vi "Lockin.DAQ.TestLauncher.vi"() -> ()   [LabVIEW 2019, in "Instrument.DAQ.lvclass"]
uses:
  Instrument.DAQ.lvclass
  <vilib>/JKI/JKI SMO/SMO/SMO.lvclass
  <vilib>/JKI/JKI SMO/SMO/Typedefs/SMOState --Enum.ctl
  Typedefs/Set State-enum.ctl
  C:/Program Files (x86)/National Instruments/LabVIEW 2019/vi.lib/JKI/JKI SMO/SMO/SMO.lvclass
  Instrument.Lockin/Instrument.Lockin.lvclass
  Instrument.Lockin/Typedefs/Results Type--Enum.ctl
  Typedefs/AO.Function--Enum.ctl
  Typedefs/AO.Channel--Cluster--Array.ctl
  Typedefs/REF.Channel--Cluster--Array.ctl
  Typedefs/DAQ.Sampling--Cluster.ctl
  Typedefs/DAQ.Sample Mode--Ring.ctl
  Typedefs/Get State-enum.ctl
  Typedefs/REF.Channel--Cluster.ctl
  Typedefs/AO.Channel--Cluster.ctl
  Typedefs/DAQ.AO.Range--enum.ctl
  Typedefs/DAQ.AI.Range--enum.ctl
  Typedefs/DAQ.AI.Coupling--enum.ctl
  Typedefs/DAQ.Configuration--Cluster.ctl
panel:
  out "DAQ state":T1=enum."created"
  in  "Tab Control 2":T2(tab)=enum."AI"
  out "AO":waveform(dbl)[](graph)
  out "AI":waveform(dbl)[](graph)
  out "WFM 3":waveform(dbl)[](graph)
  out "REF":waveform(dbl)[](graph)
  out "Results":dbl[](graph)
  in  "Reset DAQ":bool
  in  "Stop DAQ":bool
  in  "Start DAQ":bool
  in  "Tab Control":enum32{"Output", "REF", "DAQ"}(tab)=enum."REF"
  in  "Channels: AO":T3=[{"Enable?"=TRUE, "Channel"=0, "Amplitude"=0.1, "Offset"=0.0, "Frequency"=15.0, "Phase"=0.0, "Function"=enum."Sine", "Sweeping?"=FALSE}, {"Enable?"=TRUE, "Channel"=0, "Amplitude"=0.05, "Offset"=0.0, "Frequency"=13.0, "Phase"=0.0, "Function"=enum."Sine", "Sweeping?"=FALSE}] {"Phase" format="%.3g"; "Frequency" min=0.0001 max=10000.0 format="%.3g"; "Offset" format="%.3p"; "Amplitude" min=0.0 max=10.0 format="%.3p"}
  in  "Channels: Lockin":T6=[{"Enable?"=TRUE, "Channel"=1, "Frequency"=13.0, "Phase"=0.0, "TC"=1e-05, "Roll-Off"=1}] {"Roll-Off" min=1; "TC" min=0.0001 format="%#_3p"; "Phase" format="%.3g"; "Frequency" min=0.0001 max=10000.0 format="%.3g"; "Channel" min=1}
  in  "Gain":dbl[](array[numeric])=[1.0, 1.0]
  in  "sampling":T8={"Fs"=204789.0, "#s"=15753}
  in  "sample mode":T9=10123 items=["Finite Samples"=10178, "Continuous Samples"=10123]
  in  "New Ch []":T10[](array[typedef]) {"AI.Coupling" items=["AC"=10045, "DC"=10050, "GND"=10066]}
  out "SMO State":T14=enum."Stopped"
  out "error out":errorcluster
  in  "Stop":bool
  # "Basic SMO Test Launcher"
  # "For instructions on how to use the JKI State Machine Objects, examples and video tutorials, visit:\nhttp://jki.net/state-machine-objects/\n\nJKI State Machine Objects™\nhttp://jki.net/state-machine-objects/\nCopyright (C) 2005-2015, JKI <info@jki.net>\nALL RIGHTS RESERVED"
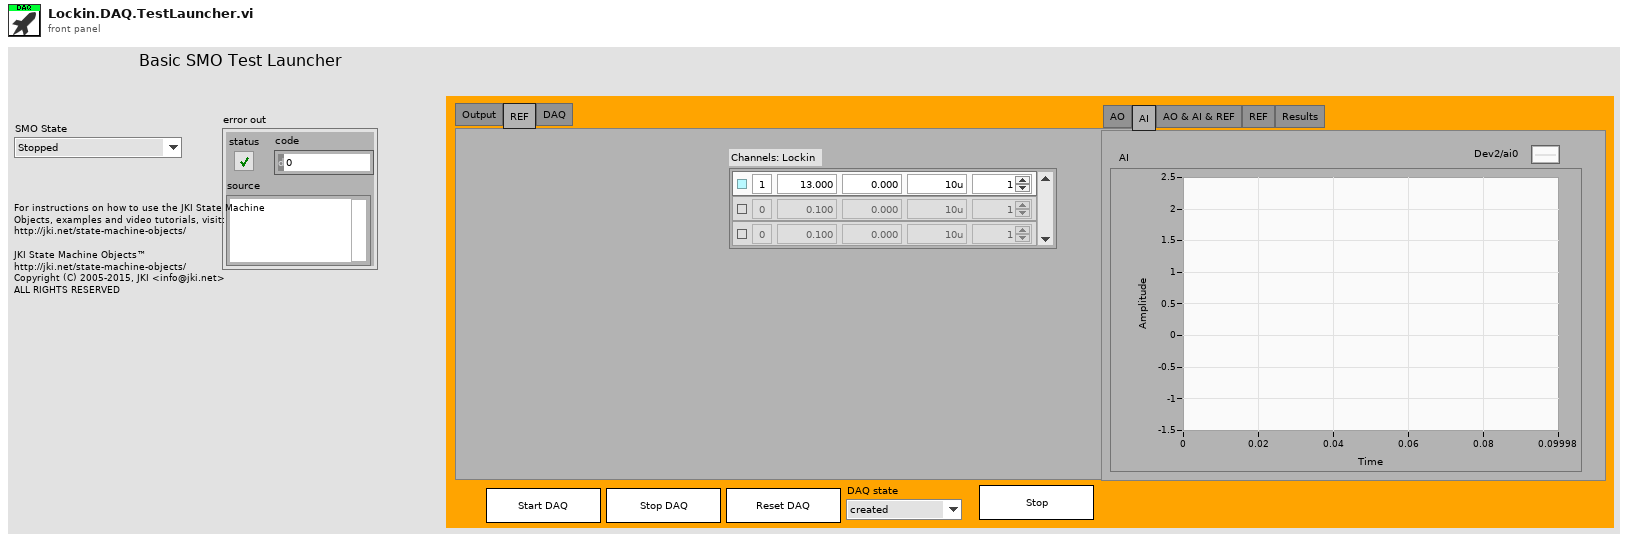
[diagram p1: front panel]
types:
  T1 = typedef "Instrument.DAQ.lvclass/Get State-enum.ctl" = enum16{"idle", "created", "started", "stopped", "sweeping"}
  T2 = enum32{"AO", "AI", "AO & AI & REF", "REF", "Results"}
  T3 = typedef "Instrument.DAQ.lvclass/AO.Channel--Cluster--Array.ctl" = T4[]
  T4 = typedef "Instrument.DAQ.lvclass/AO.Channel--Cluster.ctl" = cluster{"Enable?":bool, "Channel":i32, "Amplitude":dbl, "Offset":dbl, "Frequency":dbl, "Phase":dbl, "Function":T5, "Sweeping?":bool}
  T5 = typedef "Instrument.DAQ.lvclass/AO.Function--Enum.ctl" = enum16{"Sine", "Triangle", "Square"}
  T6 = typedef "Instrument.DAQ.lvclass/REF.Channel--Cluster--Array.ctl" = T7[]
  T7 = typedef "Instrument.DAQ.lvclass/REF.Channel--Cluster.ctl" = cluster{"Enable?":bool, "Channel":i32, "Frequency":dbl, "Phase":dbl, "TC":dbl, "Roll-Off":i32}
  T8 = typedef "Instrument.DAQ.lvclass/DAQ.Sampling--Cluster.ctl" = cluster{"Fs":dbl, "#s":i32}
  T9 = typedef "Instrument.DAQ.lvclass/DAQ.Sample Mode--Ring.ctl" = i32
  T10 = typedef "Instrument.DAQ.lvclass/DAQ.Configuration--Cluster.ctl" = cluster{"Device":string, "AO.Ch":string, "AO.Range":T11, "AI.Ch":string, "AI.Range":T12, "AI.Coupling":T13}
  T11 = typedef "Instrument.DAQ.lvclass/DAQ.AO.Range--enum.ctl" = enum16{"±0.1", "±1.0", "±10.0"}
  T12 = typedef "Instrument.DAQ.lvclass/DAQ.AI.Range--enum.ctl" = enum16{"±0.316", "±1.00", "±3.16", "±10.0", "±31.6", "±42.4"}
  T13 = typedef "Instrument.DAQ.lvclass/DAQ.AI.Coupling--enum.ctl" = u16
  T14 = typedef "SMO.lvclass/SMOState --Enum.ctl" = enum16{"unknown", "Created", "Started", "Stopped"}
  T15 = typedef "SMO.lvclass/Public Events.ctl" = cluster{"Error":refnum<user-event>, "State":refnum<user-event>, "Reserve State":refnum<user-event>}
  T16 = typedef "Instrument.DAQ.lvclass/PublicEvents--Cluster.ctl" = cluster{"getWaveforms":refnum<user-event>, "getResults":refnum<user-event>, "getCalibration":refnum<user-event>, "getAOconfig":refnum<user-event>, "getREFconfig":refnum<user-event>, "getDAQState":refnum<user-event>, "getSweepWaveforms":refnum<user-event>, "getDAQconfig":refnum<user-event>}
  T17 = cluster{"Event Registration Refnum":refnum<event-registration>}
  T18 = typedef "Instrument.DAQ.lvclass/Set State-enum.ctl" = enum16{"start", "stop", "reset", "start sweep", "stop sweep"}
  T19 = typedef "Instrument.Lockin.lvclass/Results Type--Enum.ctl" = enum16{"X", "Y", "R", "Theta", "Mean"}
  T20 = typedef "Instrument.DAQ.lvclass/DAQ.AO.config--Config--Array.ctl" = T21[]
  T21 = typedef "Instrument.DAQ.lvclass/DAQ.AO.config--Cluster.ctl" = cluster{"AO.channels":tag, "AO.Range":T11, "output terminal configuration":i32, "DAQ Type":T22}
  T22 = typedef "Instrument.DAQ.lvclass/DAQ.Type--enum.ctl" = enum16{"None", "USB 4431", "PXI 446x"}
  T23 = typedef "Instrument.DAQ.lvclass/DAQ.AI.Config--Config--Array.ctl" = T24[]
  T24 = typedef "Instrument.DAQ.lvclass/DAQ.AI.Config--Cluster.ctl" = cluster{"AI.channels":tag, "AI.Coupling":T13, "AI.Range":T12, "input terminal configuration":i32, "DAQ Type":T22}
  T25 = typedef "Instrument.DAQ.lvclass/State-enum.ctl" = enum16{"idle", "created", "started", "stopped", "sweeping"}
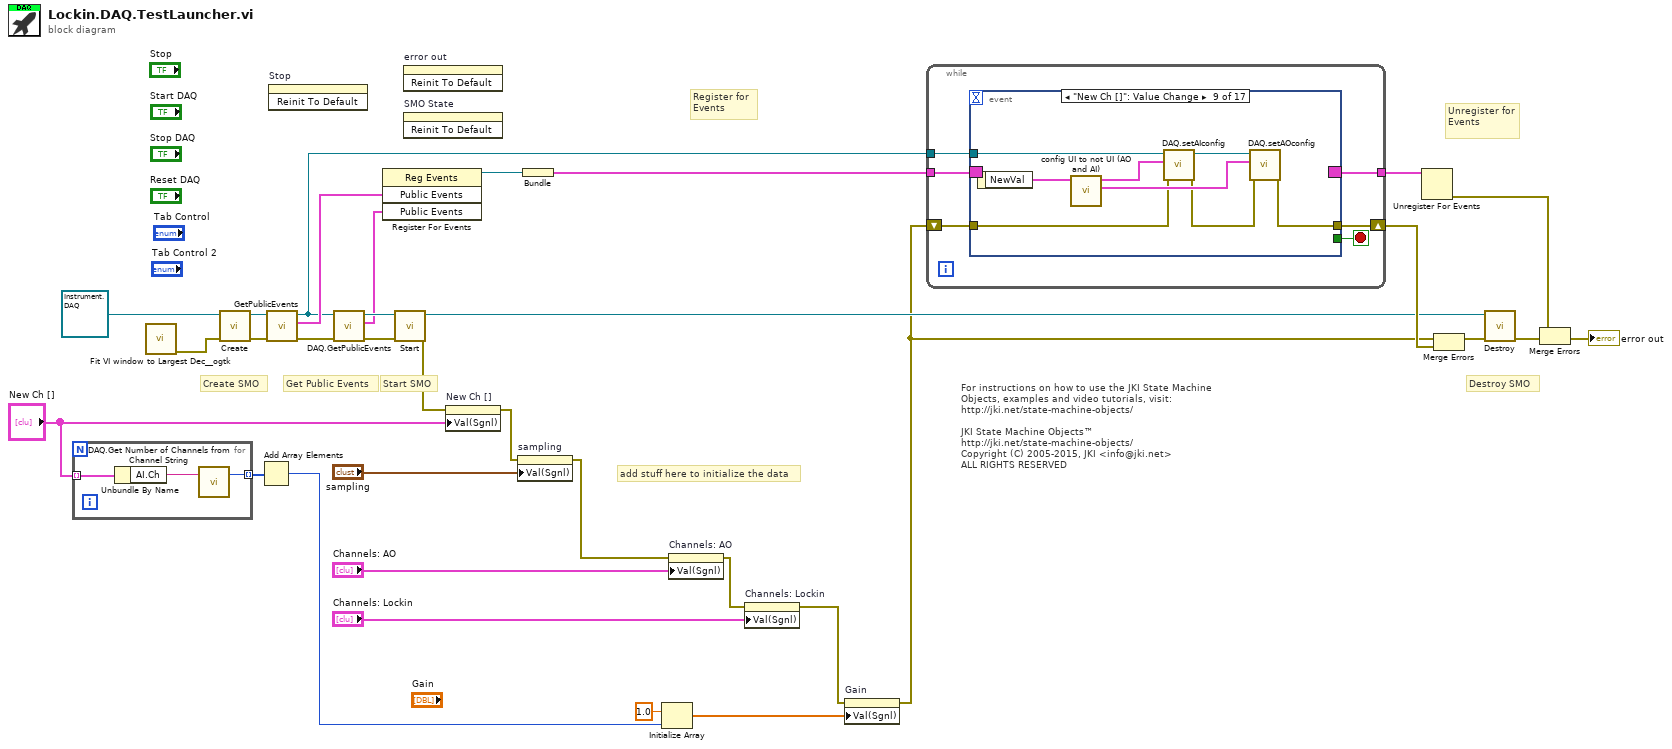
[diagram p0: block diagram]
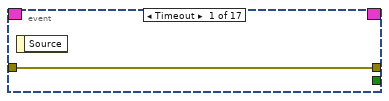
[diagram p2: hidden frame]
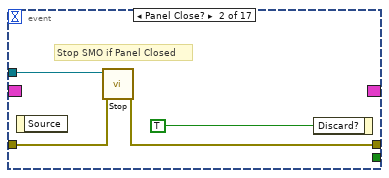
[diagram p3: hidden frame]
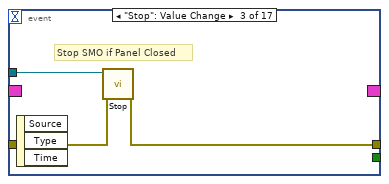
[diagram p4: hidden frame]
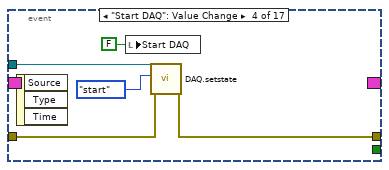
[diagram p5: hidden frame]
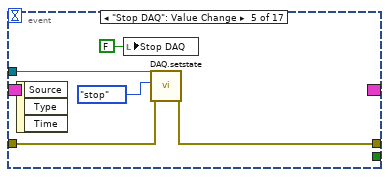
[diagram p6: hidden frame]
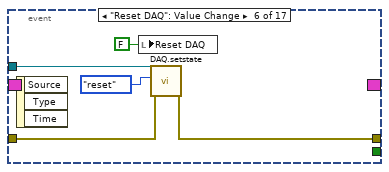
[diagram p7: hidden frame]
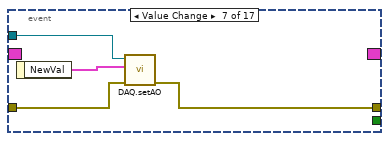
[diagram p8: hidden frame]
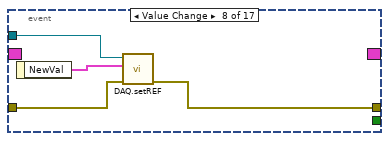
[diagram p9: hidden frame]
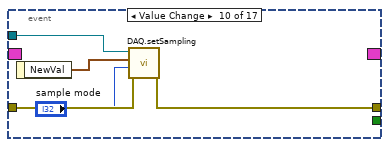
[diagram p10: hidden frame]
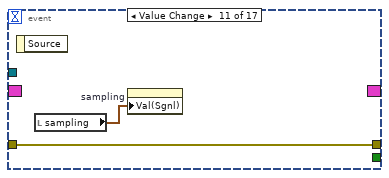
[diagram p11: hidden frame]
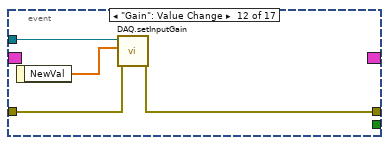
[diagram p12: hidden frame]
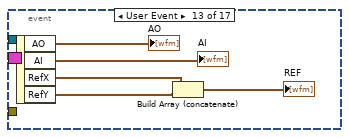
[diagram p13: hidden frame]
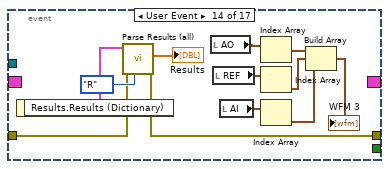
[diagram p14: hidden frame]
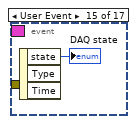
[diagram p15: hidden frame]
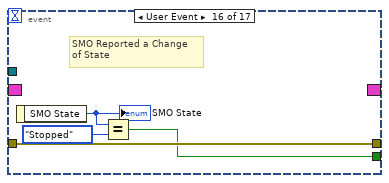
[diagram p16: hidden frame]
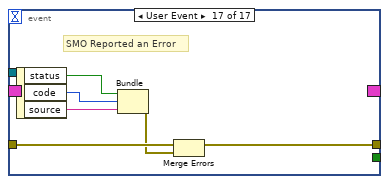
[diagram p17: hidden frame]
diagram:
  # "add stuff here to initialize the data"
  # "For instructions on how to use the JKI State Machine Objects, examples and video tutorials, visit:\nhttp://jki.net/state-machine-objects/\n\nJKI State Machine Objects™\nhttp://jki.net/state-machine-objects/\nCopyright (C) 2005-2015, JKI <info@jki.net>\nALL RIGHTS RESERVED"
  # "Get Public Events"
  # "Start SMO"
  # "Destroy SMO"
  # "Create SMO"
  # "Unregister for Events"
  # "Register for Events"
  n1 = for {
    tunnel: "New Ch []" -> [w36] mode=indexing
    tunnel: [w34] -> w12 mode=indexing
    n2 = Unbundle By Name(w36) -> ("AI.Ch"=w35:string)
    n3 = call "DAQ.Get Number of Channels from Channel String.vi"("Channels String"=w35) -> ("# channels"=w34:i32)  [unwired: 2 in]
  }
  n4 = call <userlib>:"Fit VI window to Largest Dec__ogtk.vi"() -> ("error out"=w6:errorcluster)  [unwired: 6 in, 1 out]
  n5 = call <vilib>:"Create.vi"("error in (no error)"=w6, "SMO"=refnum<class "Instrument.DAQ.lvclass"> refnum ("Lockin.DAQ.lvclass")) -> ("error out"=w25:errorcluster, "SMO out"=w26:refnum<class "Instrument.DAQ.lvclass">)  [unwired: 7 in, 1 out]
  n6 = Add Array Elements(numeric array=w12) -> (sum=w9:i32)
  n7 = call <vilib>:"GetPublicEvents.vi"("error in (no error)"=w25, "SMO"=w26) -> ("error out"=w22:errorcluster, "Public Events"=w24:T15, "SMO out"=w21:refnum<class "Instrument.DAQ.lvclass">)  [unwired: 7 in]
  n8 = invoke on="Stop" class="Bool" method="Reinit To Default"() -> ()  [unwired: 3 in, 3 out]
  n9 = call "DAQ.GetPublicEvents.vi"("error in (no error)"=w22, "Lockin.DAQ"=w21) -> ("error out"=w19:errorcluster, "Public Events"=w18:T16, "Lockin.DAQ out"=w20:refnum<class "Instrument.DAQ.lvclass">)  [unwired: 7 in]
  n10 = register-events(w24, w18) -> (reference out=w23:refnum<event-registration>)  [unwired: 2 in, 1 out]
  n11 = call <vilib>:"Start.vi"("error in (no error)"=w19, "SMO"=w20) -> ("error out"=w3:errorcluster, "SMO out"=w13:refnum<class "Instrument.DAQ.lvclass">)  [unwired: 8 in]
  n12 = invoke on="error out" class="Clust (strict)" method="Reinit To Default"() -> ()  [unwired: 3 in, 3 out]
  n13 = invoke on="SMO State" class="Enum (strict)" method="Reinit To Default"() -> ()  [unwired: 3 in, 3 out]
  n14 = property on="New Ch []" class="Arr (strict)"(error in=w3, "Val(Sgnl)"="New Ch []") -> (error out=w2:errorcluster)  [unwired: 1 in, 1 out]
  n15 = property on="sampling" class="Clust (strict)"(error in=w2, "Val(Sgnl)"="sampling") -> (error out=w1:errorcluster)  [unwired: 1 in, 1 out]
  n16 = Bundle("Event Registration Refnum"=w23) -> (w32:T17)  [unwired: 1 in]
  n17 = Initialize Array(1.0 ("element"), w9) -> (w10:dbl[])
  n18 = property on="Channels: AO" class="Arr (strict)"(error in=w1, "Val(Sgnl)"="Channels: AO") -> (error out=w14:errorcluster)  [unwired: 1 in, 1 out]
  n19 = property on="Channels: Lockin" class="Arr (strict)"(error in=w14, "Val(Sgnl)"="Channels: Lockin") -> (error out=w8:errorcluster)  [unwired: 1 in, 1 out]
  n20 = property on="Gain" class="Arr (strict)"(error in=w8, "Val(Sgnl)"=w10) -> (error out=w5:errorcluster)  [unwired: 1 in, 1 out]
  n21 = while {
    shift-right: [w41] -> w31
    shift-left: w5 -> [w40]
    tunnel: w32 -> [w39]
    tunnel: [w38] -> w33
    tunnel: w21 -> [w37]
    stop <- w42 stop-if-true
    n22 = event shown="[8] \"New Ch []\": Value Change" {
      selector: w39 -> [_ _ _ _ _ _ _ _ _ _ _ _ _ _ _ _ _]
      dyn-events: [_ _ _ _ _ _ _ _ _ _ _ _ _ _ _ _ _] -> w38
      timeout: _ -> [_ _ _ _ _ _ _ _ _ _ _ _ _ _ _ _ _]
      tunnel: [_ _ _ _ _ _ _ _ _ _ _ _ _ _ _ w111 _] -> w42
      tunnel: w37 -> [_ w47 w50 w55 w60 w65 w68 w72 w76 w86 _ w92 _ _ _ _ _]
      tunnel: [w43 w46 w49 w54 w59 w64 w66 w70 w81 w84 w87 w90 _ w98 _ w114 w118] -> w41
      tunnel: w40 -> [w43 w45 w48 w53 w58 w63 w67 w71 w74 w85 w87 w91 _ w99 _ w114 w116]
      event Timeout {
        n23 = event-data() -> ()  [unwired: 1 in, 1 out]
      }
      event Panel Close? {
        # "Stop SMO if Panel Closed"
        n24 = event-data() -> ()  [unwired: 1 in, 1 out]
        n25 = call <vilib>:"Stop.vi"("error in (no error)"=w45, "SMO"=w47) -> ("error out"=w46:errorcluster)  [unwired: 8 in, 1 out]
        n26 = event-data("Discard?"=TRUE ("OK")) -> ()  [unwired: 1 in, 1 out]
      }
      event "Stop": Value Change {
        # "Stop SMO if Panel Closed"
        n27 = event-data() -> ()  [unwired: 1 in, 3 out]
        n28 = call <vilib>:"Stop.vi"("error in (no error)"=w48, "SMO"=w50) -> ("error out"=w49:errorcluster)  [unwired: 8 in, 1 out]
      }
      event "Start DAQ": Value Change {
        n29 = event-data() -> ()  [unwired: 1 in, 3 out]
        n30 = local write "Start DAQ"(FALSE ("Start DAQ")) -> ()
        n31 = call "DAQ.setstate.vi"("error in (no error)"=w53, "State"=Set_State-enum."start" ("setState"), "Lockin.DAQ"=w55) -> ("error out"=w54:errorcluster)  [unwired: 7 in, 1 out]
      }
      event "Stop DAQ": Value Change {
        n32 = event-data() -> ()  [unwired: 1 in, 3 out]
        n33 = local write "Stop DAQ"(FALSE ("Stop DAQ")) -> ()
        n34 = call "DAQ.setstate.vi"("error in (no error)"=w58, "State"=Set_State-enum."stop" ("setState"), "Lockin.DAQ"=w60) -> ("error out"=w59:errorcluster)  [unwired: 7 in, 1 out]
      }
      event "Reset DAQ": Value Change {
        n35 = event-data() -> ()  [unwired: 1 in, 3 out]
        n36 = local write "Reset DAQ"(FALSE ("Reset DAQ")) -> ()
        n37 = call "DAQ.setstate.vi"("error in (no error)"=w63, "State"=Set_State-enum."reset" ("setState"), "Lockin.DAQ"=w65) -> ("error out"=w64:errorcluster)  [unwired: 7 in, 1 out]
      }
      event Value Change {
        n38 = event-data() -> ("NewVal"=w69:T3)  [unwired: 1 in]
        n39 = call "DAQ.setAO.vi"("error in (no error)"=w67, "AO Channels"=w69, "Lockin.DAQ"=w68) -> ("error out"=w66:errorcluster)  [unwired: 7 in, 1 out]
      }
      event Value Change {
        n40 = event-data() -> ("NewVal"=w73:T6)  [unwired: 1 in]
        n41 = call "DAQ.setREF.vi"("error in (no error)"=w71, "Channels: Lockin"=w73, "Lockin.DAQ"=w72) -> ("error out"=w70:errorcluster)  [unwired: 7 in, 1 out]
      }
      event "New Ch []": Value Change {
        n42 = event-data() -> ("NewVal"=w80:T10[])  [unwired: 1 in]
        n43 = call "config UI to not UI (AO and AI).vi"("New Ch []"=w80) -> ("AO Config"=w78:T20, "AI Config"=w79:T23)  [unwired: 9 in]
        n44 = call "DAQ.setAIconfig.vi"("error in (no error)"=w74, "AI Configuration"=w79, "Lockin.DAQ"=w76) -> ("error out"=w75:errorcluster, "Lockin.DAQ out"=w77:refnum<class "Instrument.DAQ.lvclass">)  [unwired: 7 in]
        n45 = call "DAQ.setAOconfig.vi"("error in (no error)"=w75, "AO Configuration"=w78, "Lockin.DAQ"=w77) -> ("error out"=w81:errorcluster)  [unwired: 7 in, 1 out]
      }
      event Value Change {
        n46 = event-data() -> ("NewVal"=w83:T8)  [unwired: 1 in]
        n47 = call "DAQ.setSampling.vi"("error in (no error)"=w85, "Sample Mode"="sample mode", "Sampling"=w83, "Lockin.DAQ"=w86) -> ("error out"=w84:errorcluster)  [unwired: 6 in, 1 out]
      }
      event Value Change {
        n48 = event-data() -> ()  [unwired: 1 in, 1 out]
        n49 = local read "sampling"() -> (w88:T8)
        n50 = property on="sampling" class="Clust (strict)"("Val(Sgnl)"=w88) -> ()  [unwired: 2 in, 2 out]
      }
      event "Gain": Value Change {
        n51 = event-data() -> ("NewVal"=w89:dbl[])  [unwired: 1 in]
        n52 = call "DAQ.setInputGain.vi"("error in (no error)"=w91, "setInputGain"=w89, "Lockin.DAQ"=w92) -> ("error out"=w90:errorcluster)  [unwired: 7 in, 1 out]
      }
      event User Event {
        n53 = event-data() -> ("AO"=→"AO":waveform(dbl)[], "AI"=→"AI":waveform(dbl)[], "RefX"=w95:waveform(dbl)[], "RefY"=w94:waveform(dbl)[])  [unwired: 1 in]
        n54 = Build Array (concatenate)(w95, w94) -> (→"REF":waveform(dbl)[])
      }
      event User Event {
        n55 = event-data() -> ("Results.Results (Dictionary)"=w102:cluster{"key":string, "value":dbl}[])  [unwired: 1 in]
        n56 = call "Parse Results (all).vi"("Type"=Results_Type--Enum."R", "error in (no error)"=w99, "Results (Dictionary)"=w102) -> ("error out"=w98:errorcluster, "Data"=→"Results":dbl[])  [unwired: 5 in, 2 out]
        n57 = local read "AO"() -> (w109:waveform(dbl)[])
        n58 = local read "REF"() -> (w108:waveform(dbl)[])
        n59 = local read "AI"() -> (w107:waveform(dbl)[])
        n60 = Index Array(array=w109) -> (element=w106:waveform(dbl))  [unwired: 1 in]
        n61 = Index Array(array=w108) -> (element=w105:waveform(dbl))  [unwired: 1 in]
        n62 = Index Array(array=w107) -> (element=w103:waveform(dbl))  [unwired: 1 in]
        n63 = Build Array(w106, w105, w103) -> (→"WFM 3":waveform(dbl)[])
      }
      event User Event {
        n64 = event-data() -> ("state"=→"DAQ state":T25)  [unwired: 1 in, 2 out]
      }
      event User Event {
        # "SMO Reported a Change\nof State"
        n65 = event-data() -> ("SMO State"=w113:T14)  [unwired: 1 in]
        "SMO State" <- w113
        n66 = Equal?(x=w113, y=SMOState_--Enum."Stopped") -> (x = y?=w111:bool)
      }
      event User Event {
        # "SMO Reported an Error"
        n67 = event-data() -> ("status"=w117:bool, "code"=w120:i32, "source"=w119:string)  [unwired: 1 in]
        n68 = Bundle("status"=w117, "code"=w120, "source"=w119) -> (w115:errorcluster)  [unwired: 1 in]
        n69 = Merge Errors(w116, w115) -> (w118:errorcluster)
      }
    }
  }
  n70 = Unregister For Events(event registration refnum=w33) -> (error out=w30:errorcluster)  [unwired: 1 in]
  n71 = Merge Errors(w5, w31) -> (w27:errorcluster)
  n72 = call <vilib>:"Destroy.vi"("error in (no error)"=w27, "SMO"=w13) -> ("error out"=w28:errorcluster)  [unwired: 9 in]
  n73 = Merge Errors(w30, w28) -> (→"error out":errorcluster)
